vi "DAC Configure.vi"(8 "error in":errorcluster, 11 "DAC TC Temperature in":refnum<class "DAC TC Temp DeepU.lvclass">) -> (0 "error out":errorcluster, 3 "DAC TC Temperature out":refnum<class "DAC TC Temp DeepU.lvclass">)   [LabVIEW 2019, in "DAC.lvlib" / "DAC TC Temp DeepU.lvclass"]
uses:
  DAC TC Temp DeepU.lvclass
  C:/Users/krio/Documents/LV_Projects/test-stand/App/DAC/DAC.lvclass
  DAC.lvclass/DAC.ctl
  DAC TC Temp DeepU.lvclass/DAC TC Temp DeepU.ctl
  <vilib>/DAQmx/create/channels.llb/DAQmx Create Channel (AI-Temperature-Thermocouple).vi
  DAC.lvclass
  <resource>/objmgr/daqmx.rc
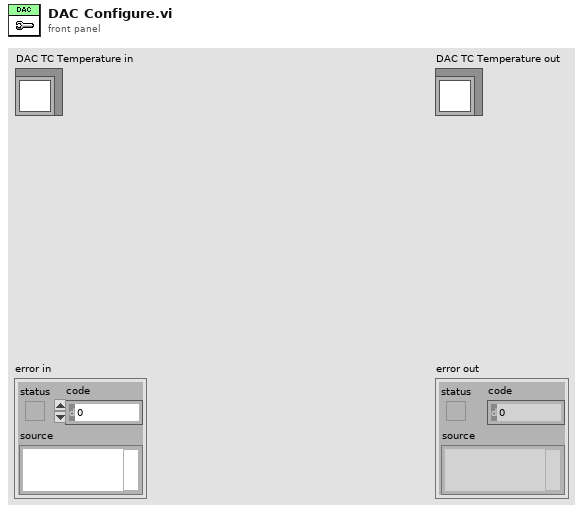
[diagram p1: front panel]
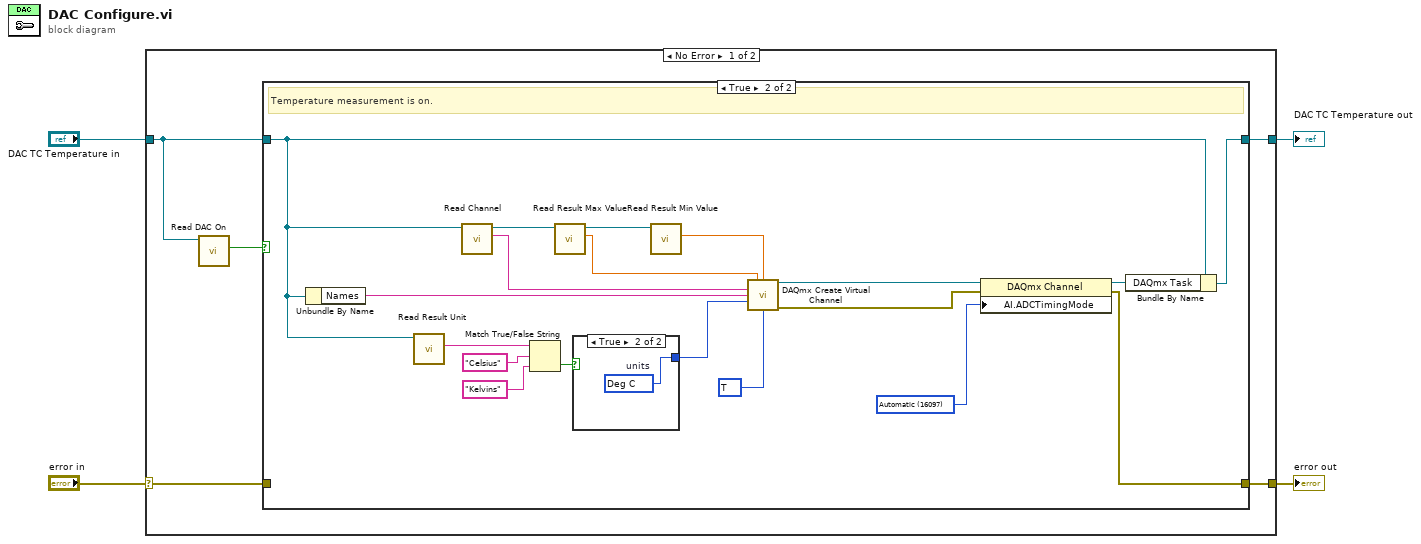
[diagram p0: block diagram]
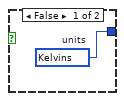
[diagram p3: hidden frame]
diagram:
  n1 = case shown="No Error" "error in" {
    selector: "error in" -> [w6 w34]
    tunnel: [w5 w34] -> w4
    tunnel: [w7 w33] -> w3
    tunnel: "DAC TC Temperature in" -> [w9 w33]
    frame No Error {
      n2 = call "Read DAC On.vi"("DAC in"=w9) -> ("DAC On"=w8:bool)  [unwired: 8 in, 2 out]
      n3 = case shown="True" w8 {
        tunnel: w9 -> [w11 w20]
        tunnel: [w11 w26] -> w7
        tunnel: w6 -> [w10 _]
        tunnel: [w10 w13] -> w5
        frame False {
          # "Temperature measurement is off."
        }
        frame True {
          w12 = 10086 items=["J"=10072, "K"=10073, "N"=10077, "R"=10082, "S"=10085, "T"=10086, "B"=10047, "E"=10055] ("thermocouple type")
          w22 = 16097 items=["Automatic"=16097, "High Resolution"=10195, "High Speed"=14712, "Best 50 Hz Rejection"=14713, "Best 60 Hz Rejection"=14714, "Custom"=10137] ("AI.ADCTimingMode")
          # "Temperature measurement is on."
          n4 = Unbundle By Name(w20) -> ("Names"=w25:string)
          n5 = call "Read Result Unit.vi"("DAC in"=w20) -> ("Unit"=w21:string)  [unwired: 8 in, 2 out]
          n6 = call "Read Channel.vi"("DAC in"=w20) -> ("Channel"=w19:string, "DAC out"=w18:refnum<class "DAC TC Temp DeepU.lvclass">)  [unwired: 8 in, 1 out]
          n7 = Match True/False String(2:"Kelvins" ("false string"), 3:"Celsius" ("true string"), 4:w21) -> (0:w28:bool)  [unwired: 1 out]
          n8 = call "Read Result Max Value.vi"("DAC in"=w18) -> ("Max Value"=w15:dbl, "DAC out"=w17:refnum<class "DAC TC Temp DeepU.lvclass">)  [unwired: 8 in, 1 out]
          n9 = case shown="True" w28 {
            tunnel: [w31 w32] -> w27
            frame False {
              w31 = 10325 items=["Deg C"=10143, "Deg F"=10144, "Kelvins"=10325, "Deg R"=10145, "From Custom Scale"=10065]  # units
            }
            frame True {
              w32 = 10143 items=["Deg C"=10143, "Deg F"=10144, "Kelvins"=10325, "Deg R"=10145, "From Custom Scale"=10065]  # units
            }
          }
          n10 = call "Read Result Min Value.vi"("DAC in"=w17) -> ("Min Value"=w16:dbl)  [unwired: 8 in, 2 out]
          n11 = call-poly <vilib>:"DAQmx Create Virtual Channel.vi"("maximum value"=w15, "minimum value"=w16, "physical channels"=w19, "name to assign"=w25, "units"=w27, "thermocouple type"=w12) -> ("task out"=w24:refnum<k21>, "error out"=w14:errorcluster)  [unwired: 8 in]
          n12 = property class="DAQmx Channel"(reference=w24, error in=w14, "AI.ADCTimingMode"=w22) -> (reference out=w23:refnum<k21>, error out=w13:errorcluster)
          n13 = Bundle By Name(cluster=w20, "DAQmx Task"=w23) -> (w26:refnum<class "DAC TC Temp DeepU.lvclass">)
        }
      }
    }
    frame Error {
    }
  }
  "error out" <- w4
  "DAC TC Temperature out" <- w3
